vi "Where I Am.vi"() -> ()   [LabVIEW 2010]
uses:
  6-OCU Neurons/MDF LatLong.ctl
  5.0-Global.vi
panel:
  out "Where?":bool
  out "5.1.1 MDF GPS Out":T1[](array[typedef])
  out "5.1.1 MDF XY Out":T1[](array[typedef])
  out "XY Graph":cluster{ext[], ext[]}(graph)
  out "Array of GPS coors":ext[][](array[numeric])
  # "Update MDF - XY"
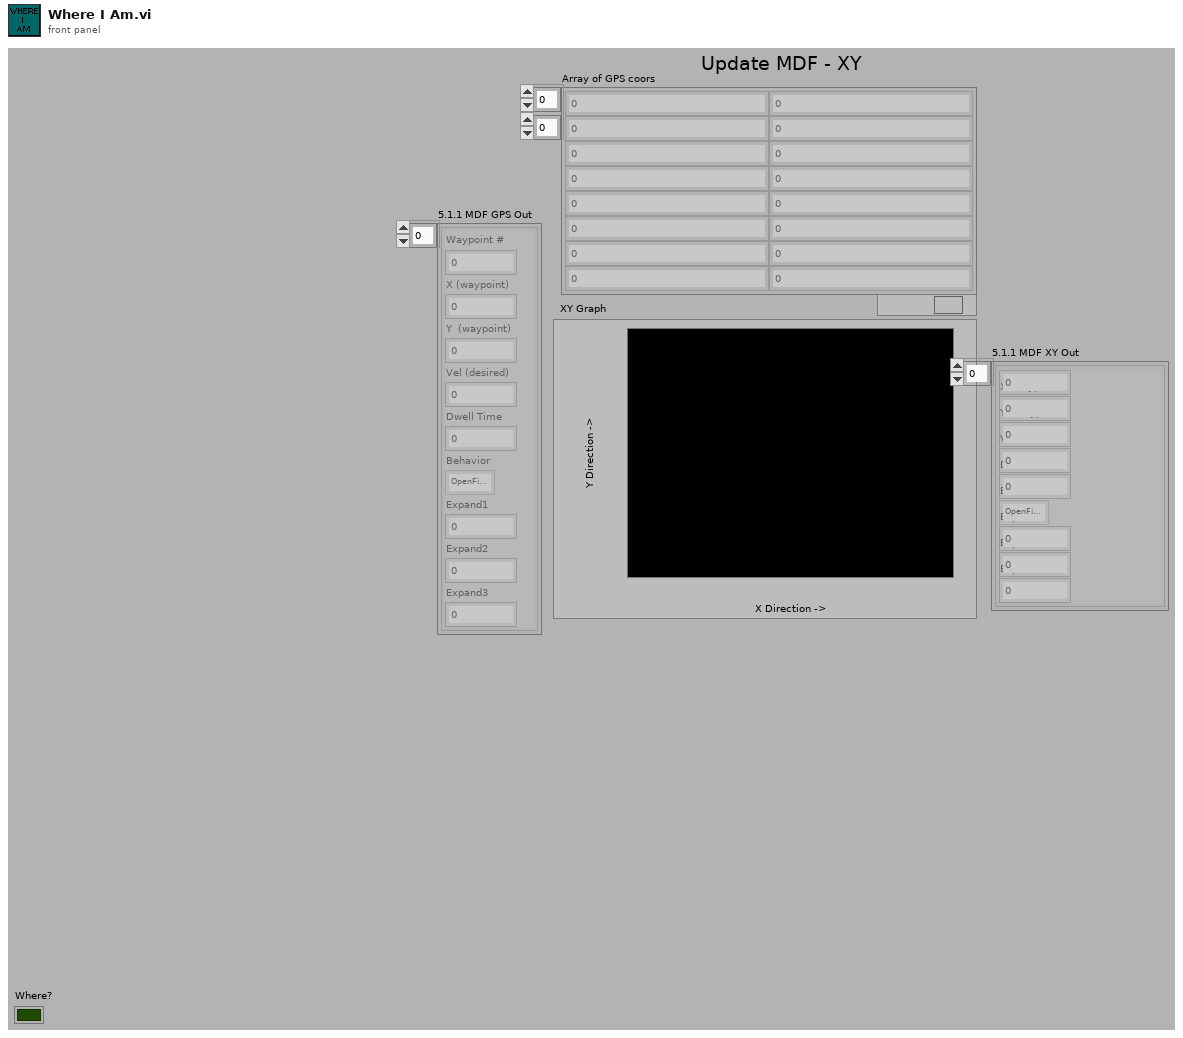
[diagram p1: front panel]
types:
  T1 = typedef "MDF LatLong.ctl" = cluster{"Waypoint #":dbl, "X (waypoint)":ext, "Y  (waypoint)":ext, "Vel (desired)":dbl, "Dwell Time":dbl, "Behavior":enum16{"OpenFieldTransit", "WallFollow", "LaneFollow", "ManualMode"}, "Expand1":dbl, "Expand2":dbl, "Expand3":dbl}
  T2 = cluster{"Waypoint #":bool, "X (waypoint)":bool, "Y  (waypoint)":bool, "Vel (desired)":bool, "Dwell Time":bool, "Behavior":bool, "Expand1":bool, "Expand2":bool, "Expand3":bool}[]
  T3 = cluster{"Waypoint #":bool, "X (waypoint)":bool, "Y  (waypoint)":bool, "Vel (desired)":bool, "Dwell Time":bool, "Behavior":bool, "Expand1":bool, "Expand2":bool, "Expand3":bool}
  T4 = typedef "MDF XY.ctl" = T1[]
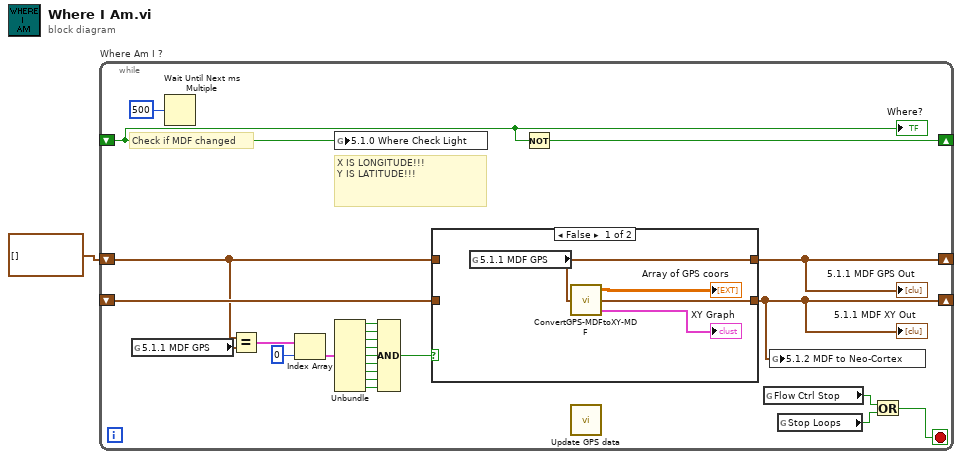
[diagram p0: block diagram]
diagram:
  n1 = while "Where Am I ?" {
    shift-right: [w24] -> _
    shift-left: _ -> [w23]
    shift-right: [w5] -> _
    shift-left: T1[] [] ("5.1.1 MDF GPS Out 2") -> [w7]
    shift-right: [w6] -> _
    shift-left: _ -> [w8]
    stop <- w2 stop-if-true
    # "Check if MDF changed"
    # "X IS LONGITUDE!!!\nY IS LATITUDE!!!"
    n2 = global read "5.0-Global.vi" "5.1.1 MDF GPS"() -> (w22:T1[])
    n3 = Wait Until Next ms Multiple(millisecond multiple=u32 500 ("milliseconds to wait")) -> ()  [unwired: 1 out]
    n4 = Equal?(x=w7, y=w22) -> (x = y?=w9:T2)
    n5 = Index Array(array=w9, index=0) -> (element=w12:T3)
    n6 = global write "5.0-Global.vi" "5.1.0 Where Check Light"(w23) -> ()
    n7 = Unbundle(w12) -> ("Waypoint #"=w13:bool, "X (waypoint)"=w14:bool, "Y  (waypoint)"=w15:bool, "Vel (desired)"=w16:bool, "Dwell Time"=w17:bool, "Behavior"=w18:bool, "Expand1"=w19:bool, "Expand2"=w20:bool, "Expand3"=w21:bool)
    n8 = Compound Arithmetic op=AND(w13, w14, w15, w16, w17, w18, w19, w20, w21) -> (w11:bool)
    n9 = case shown="False" w11 {
      tunnel: w7 -> [_ w31]
      tunnel: [w26 w31] -> w5
      tunnel: [w29 w30] -> w6
      tunnel: w8 -> [_ w30]
      frame False {
        n10 = global read "5.0-Global.vi" "5.1.1 MDF GPS"() -> (w26:T1[])
        n11 = call "ConvertGPS-MDFtoXY-MDF.vi"("5.1.1 MDF GPS"=w26) -> ("XY Graph"=→"XY Graph":cluster{ext[], ext[]}, "5.1.1 MDF XY"=w29:T4, "Array of GPS coors"=→"Array of GPS coors":ext[][])
      }
      frame True {
      }
    }
    "5.1.1 MDF XY Out" <- w6
    "5.1.1 MDF GPS Out" <- w5
    n12 = Not(x=w23) -> (.not. x?=w24:bool)
    n13 = call "Update GPS data.vi"() -> ()  [unwired: 12 in]
    n14 = global read "5.0-Global.vi" "Flow Ctrl Stop"() -> (w4:bool)
    n15 = global write "5.0-Global.vi" "5.1.2 MDF to Neo-Cortex"(w6) -> ()
    n16 = global read "5.0-Global.vi" "Stop Loops"() -> (w3:bool)
    n17 = Or(x=w4, y=w3) -> (x .or. y?=w2:bool)
    "Where?" <- w23
  }
